vi "SCMP - Externally Triggered Image Acquisition - v5.vi"(0 "FPS":dbl=10.0 format="%.1g", 1 "LCVR Voltages":dbl[][](array[numeric]), 2 "Mod/Seq":bool, 5 "Cycles":i32=1 min=1 max=30 step=1, 7 "Save to FITS?":bool=TRUE, 9 "Headers In":T12[](array[typedef])=[{"Wavelength (nm)"=530.15, "Exposure (s)"=0.05, "Tuning Delay (ms)"=1000.0, "Beam Type (-1/1)"=1.0, "Tuning Voltages"=[1.111, 2.222, 3.333, 4.444], "Observer"="observer", "Light Shapping Diffuser"=enum."In Beam", "Comment"="", "Data Type"=9, "Mod Cycles"=0, "SCD Calibration Optics"=enum."1 - Polarizer @0, I+Q", "SCD Emission Line Filter"=enum."1-557.6nm", "Cookbook"="", "COMP-S Calibration Wheel"=enum."Dark", "COMP-S Andover Filter Wheel"=enum."530.3nm/HWB 0.34nm (Fe XIV)", "FOV Rotation (deg)"=66.0, "Objective Lens Position (mm)"=0.0, "Occulter size"=0.0, "Time End"=timestamp(3382374145.421875 s since 1904-01-01), "Acc Exposure (s)"=0.0, "Time Stamp Array"=[], "Camera Serial Number"=[], "Camera Temp"=[], "Camera PI (mm)"=[], "Time Start"=timestamp(3382374145.421875 s since 1904-01-01), "Peripherals"={"ILX controler"=FALSE, "Zone temperatures"=FALSE, "Andor"=FALSE, "Andor 2"=FALSE, "PI Stages"=FALSE, "AISAS mechanisms"=FALSE, "AISAS Mech.lvclass"=refnum, "Zone temp ref"=variant, "FWs"=FALSE}, "FITS paths"=[], "Cameras"=enum."Andor", "load preset cbk"=FALSE, "periodic check count"=0, "COMP-S Calibration Wheel 2"=enum."Dark", "Calib"=enum."Dark", "Abso Aperture"=40.0, "Nominal Aperture"=196.0}] {"Nominal Aperture" format="%.1f"; "Abso Aperture" format="%.1f"; "Camera PI (mm)" format="%_3g"; "Acc Exposure (s)" format="%^.3g"; "Occulter size" format="%.2f"; "Objective Lens Position (mm)" min=70.0 max=152.0 format="%.2f"; "FOV Rotation (deg)" format="%.1f"; "Data Type" items=["LIVE", "DARK", "FLAT", "CALI", "OBSE", "ABSO", "AURE", "TARG", "OBJE", "HOLE", "OREX", "THRO", "CHIP"]; "Exposure (s)" format="%^.3g"; "Wavelength (nm)" format="%_6g"}, 11 "error in":errorcluster, 12 "Andor Neo":T13[](array[typedef]) {"Exposure (s)" format="%^.3g"; "Time at Synch" format="%<%H:%M:%S>T"; "Interframe Time" format="%#_3g"; "Frame Readout Time" format="%_3g"; "Row Readout Time" format="%_3g"}) -> (3 "FITS Path Out":path, 6 "Image":u32[][](array[numeric]), 8 "Camera R Image":u32[][](graph), 10 "Headers Out":T2[](array[typedef]) {"Nominal Aperture" format="%.1f"; "Abso Aperture" format="%.1f"; "Camera PI (mm)" format="%_3g"; "Acc Exposure (s)" format="%^.3g"; "Occulter size" format="%.2f"; "Objective Lens Position (mm)" min=70.0 max=152.0 format="%.2f"; "FOV Rotation (deg)" format="%.1f"; "Exposure (s)" format="%^.3g"; "Wavelength (nm)" format="%_6g"}, 13 "FITS Path Out 2":path, 14 "Break":bool, 15 "error out":errorcluster)   [LabVIEW 2014]
doc: "The LL Sequence VI acquires a sequence of images and displays them in an array of image controls using the low-level acquisition VIs. A sequence is appropriate for applications that process multiple images. You can configure a sequence to acquire every frame or to skip a variable number of frames between each image.\n\nTop Level Code Overview\n1) Initialize Camera (Global Shutter, High Well, Low Noise, exposure time, etc.)\n2) Create a buffer set equal in size to the # of trigger pulses (e.g. 100) which is the same as the # of expected images \n3) Start the camera acquisition THEN start the DAQmx task (use merge error cluster to gurantee this)"
uses:
  Camera/Andor Neo Info.ctl
  Controls/run cbk timeout.ctl
  <vilib>/Waveform/WDTOps.llb/WDT Waveform Duration DBL.vi
  <vilib>/DAQmx/write.llb/DAQmx Write (Analog 1D Wfm NChan NSamp).vi
  <vilib>/DAQmx/create/channels.llb/DAQmx Create Channel (AO-Voltage-Basic).vi
  <vilib>/DAQmx/configure/timing.llb/DAQmx Timing (Use Waveform).vi
  Controls/Global demo.vi
  Controls/beaning.ctl
  Controls/SCD - Calibration Optics Filter Wheel.ctl
  AISAS/Controls/Diffuser.ctl
  Controls/SCD - FITS Cluster.ctl
  Controls/SCD - EDT - Emission Line Filter Wheel.ctl
  Controls/CoMP-S Controls/Polarization Optics Filter Wheel.ctl
  Controls/CoMP-S Controls/Emission Line Filter Wheel.ctl
  AISAS/Controls/focus.ctl
  AISAS/Mech/AISAS Mech.lvclass
  Controls/peripherals.ctl
  Controls/Cameras select.ctl
  Controls/FITS Data type.ctl
panel:
  out "Break 2":bool
  out "display refresh":bool
  out "seq cycles":i32=1
  out "error dequeue RAM":errorcluster
  out "mod cycles *4":i32=1
  out "error cam dequeue & queue RAM":errorcluster
  out "error dequeue 2":errorcluster
  in  "count 2":i32
  in  "Tab Control":T1(tab)
  out "Camera T Image":u32[][](graph)
  out "# elements in RAM queue":i32
  out "Image Acq (s)":dbl(slide)=4151.832132564842
  out "Image SSD Saving":i32(slide) scale=0.0..1.0
  in  "user break":bool
  out "Camera T Image wide":u32[][](graph)
  out "# images to acquire":i32
  out "Image Acq Started":bool
  out "PixelData [U16]":u16[](array[numeric])
  out "ByteData [U8]":u8[](array[numeric])
  in  "image pointers":u64[](array[numeric])
  in  "imageNo":i32
  in  "count":i32
  out "# wavelengths":i32=1
  out "Exposure Get (s)":dbl=0.09 format="%_3p"
  out "# elements in queue":i32
  out "Image Cam":u32[][](graph)
  out "# buffer":i32
  in  "image pointers 2":u64[](array[numeric])
  in  "imageNo 2":i32
  out "# elements in queue 2":i32
  out "# buffer 2":i32
  out "Image transfering":u32(slide) scale=0.0..40.0
  out "Acquisition Estimate (s)":dbl format="%0.2f"
  out "Image Acq":i32(slide) scale=0.0..40.0
  out "Image Acq 2":i32(slide) scale=0.0..40.0
  out "Image SSD Saving 2":i32(slide) scale=0.0..1.0
  out "Time Start":timestamp=timestamp(3382374145.421875 s since 1904-01-01) format="%<%H:%M:%S%3u\n%x>T"
  out "Time stamp arr":timestamp[](array[timestamp]) format="%<%H:%M:%S%3u>T"
  out "COMP Waveforms":waveform(dbl)[](graph)
  out "SCD Waveforms":waveform(dbl)[](graph)
  out "Time stamp arr 2":timestamp[](array[timestamp]) format="%<%H:%M:%S%3u>T"
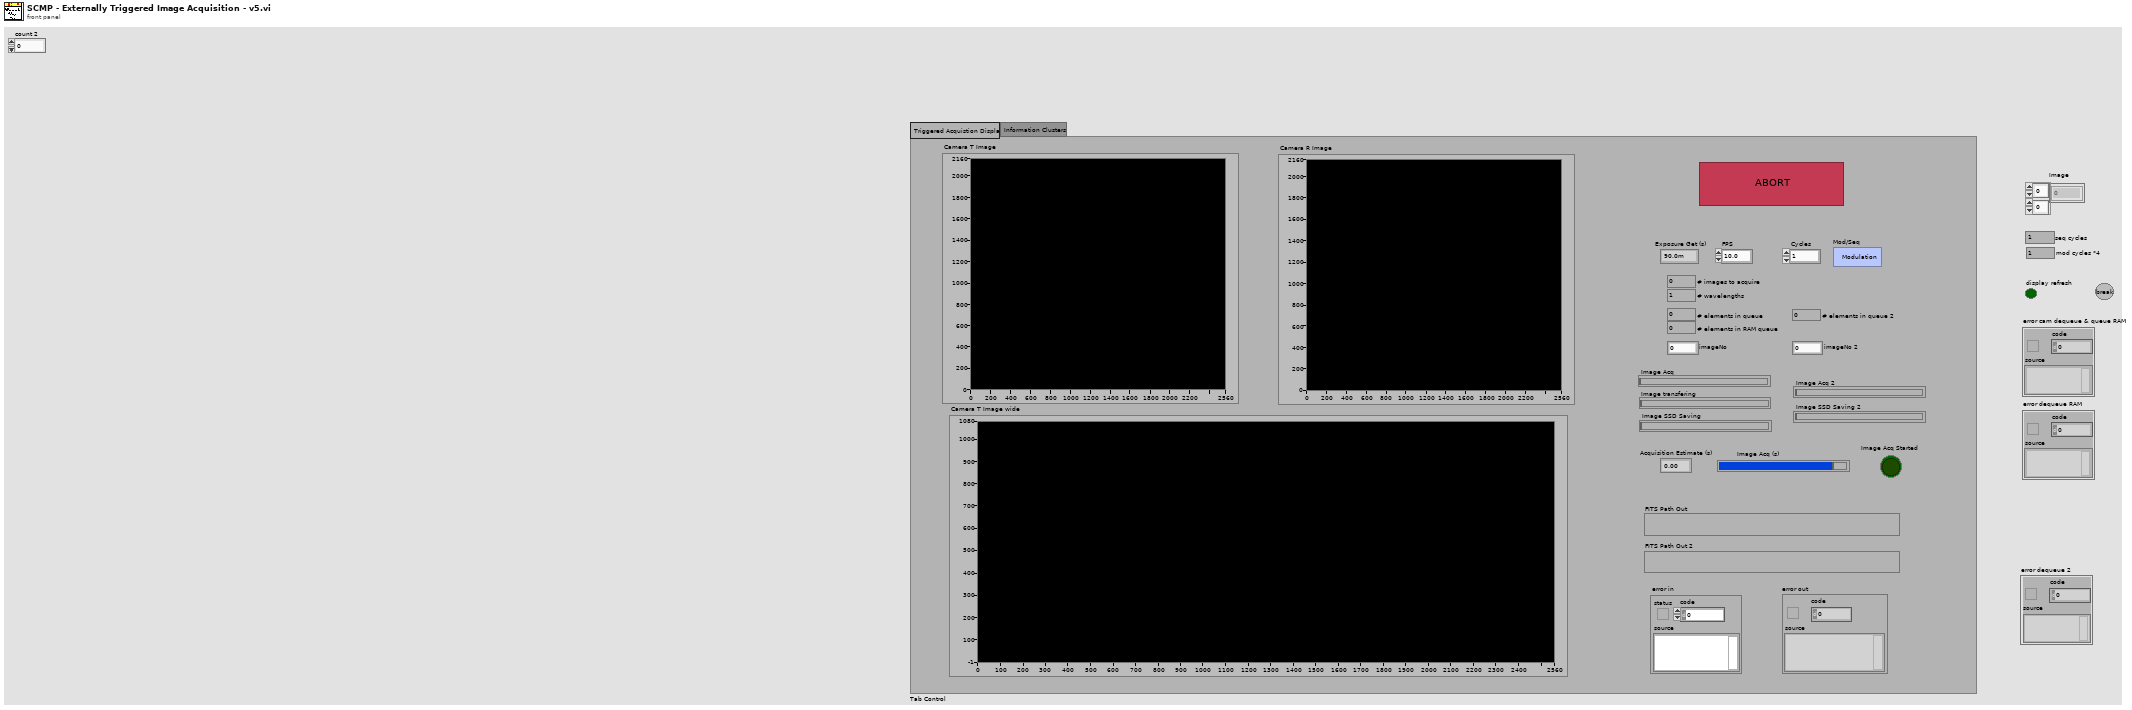
[diagram p1: front panel]
types:
  T1 = enum32{"Triggered Acquistion Display", "Information Clusters"}
  T2 = typedef "SCD - FITS Cluster.ctl" = cluster{"Wavelength (nm)":dbl, "Exposure (s)":dbl, "Tuning Delay (ms)":dbl, "Beam Type (-1/1)":dbl, "Tuning Voltages":dbl[], "Observer":string, "Light Shapping Diffuser":T3, "Comment":string, "Data Type":T4, "Mod Cycles":u16, "SCD Calibration Optics":T5, "SCD Emission Line Filter":T6, "Cookbook":string, "COMP-S Calibration Wheel":T7, "COMP-S Andover Filter Wheel":T8, "FOV Rotation (deg)":dbl, "Objective Lens Position (mm)":T9, "Occulter size":dbl, "Time End":timestamp, "Acc Exposure (s)":dbl, "Time Stamp Array":timestamp[], "Camera Serial Number":string[], "Camera Temp":dbl[], "Camera PI (mm)":dbl[], "Time Start":timestamp, "Peripherals":T10, "FITS paths":path[], "Cameras":T11, "load preset cbk":bool, "periodic check count":i32, "COMP-S Calibration Wheel 2":T7, "Calib":enum16{"Dark", "Flat"}, "Abso Aperture":dbl, "Nominal Aperture":dbl, "Pointer IP":string}
  T3 = typedef "Diffuser.ctl" = enum16{"Out of Beam", "In Beam"}
  T4 = typedef "FITS Data type.ctl" = enum16{"LIVE", "DARK", "FLAT", "CALI", "OBSE", "ABSO", "AURE", "TARG", "OBJE", "HOLE", "OREX", "THRO", "CHIP"}
  T5 = typedef "SCD - Calibration Optics Filter Wheel.ctl" = enum16{"1 - Polarizer @0, I+Q", "2 - Polarizer @90, I-Q", "3 - Polarizer @45, I+U", "4 - Polarizer @135, I-U", "5 - Polarizer @0, Retarder @45, I+V", "6 - Polarizer @0, Retarder @135, I-V", "7 - Dark", "8 - Clear", "9 - N/A"}
  T6 = typedef "SCD - EDT - Emission Line Filter Wheel.ctl" = enum16{"1-557.6nm", "2-587.6nm", "3-589.6nm", "4-630.2nm", "5-656.4nm", "6-849.8nm", "7-854.2nm", "8-866.2nm", "9-1083.0nm"}
  T7 = typedef "Polarization Optics Filter Wheel.ctl" = enum16{"Dark", "Clear", "Exchange Lens", "Polarizer @0, I+Q", "Polarizer @90, I-Q", "Polarizer @45, I+U", "Polarizer @135, I-U", "Polarizer @0, Retarder @45, I+V", "Polarizer @0, Retarder @135, I-V"}
  T8 = typedef "Emission Line Filter Wheel.ctl" = enum16{"530.3nm/HWB 0.34nm (Fe XIV)", "587.6nm/HBW 0.44nm (He I D3)", "637.5nm/HBW 0.53nm (Fe X)", "656.3nm/HBW 0.57nm (H-Alpha)", "789.2nm/HBW 0.85nm (Fe XI)", "854.2nm/HBW 1.01nm (Ca I)", "1074.7nm/HBW 2.34nm (Fe XIII)", "1079.8nm/HBW 1.64nm (Fe XIII)", "1083.0nm/HBW 1.66nm (He I)"}
  T9 = typedef "focus.ctl" = dbl
  T10 = typedef "peripherals.ctl" = cluster{"ILX controler":bool, "Zone temperatures":bool, "Andor":bool, "Andor 2":bool, "PI Stages":bool, "AISAS mechanisms":bool, "AISAS Mech.lvclass":refnum<class "AISAS Mech.lvclass">, "Zone temp ref":variant, "FWs":bool}
  T11 = typedef "Cameras select.ctl" = enum16{"Andor", "GDR"}
  T12 = typedef "SCD - FITS Cluster.ctl" = cluster{"Wavelength (nm)":dbl, "Exposure (s)":dbl, "Tuning Delay (ms)":dbl, "Beam Type (-1/1)":dbl, "Tuning Voltages":dbl[], "Observer":string, "Light Shapping Diffuser":T3, "Comment":string, "Data Type":u16, "Mod Cycles":u16, "SCD Calibration Optics":T5, "SCD Emission Line Filter":T6, "Cookbook":string, "COMP-S Calibration Wheel":T7, "COMP-S Andover Filter Wheel":T8, "FOV Rotation (deg)":dbl, "Objective Lens Position (mm)":T9, "Occulter size":dbl, "Time End":timestamp, "Acc Exposure (s)":dbl, "Time Stamp Array":timestamp[], "Camera Serial Number":string[], "Camera Temp":dbl[], "Camera PI (mm)":dbl[], "Time Start":timestamp, "Peripherals":T10, "FITS paths":path[], "Cameras":T11, "load preset cbk":bool, "periodic check count":i32, "COMP-S Calibration Wheel 2":T7, "Calib":enum16{"Dark", "Flat"}, "Abso Aperture":dbl, "Nominal Aperture":dbl}
  T13 = typedef "Andor Neo Info.ctl" = cluster{"Handle":i32, "Pixel Encoding":string, "AOI Width":i32, "AOI Height":i32, "AOI Stride":i32, "Row Readout Time":dbl, "Frame Readout Time":dbl, "Interframe Time":dbl, "Semaphore":T14, "SerialNumber":string, "Camera Model":string, "Controller ID":string, "Firmware Version":string, "Shutter":string, "BDiv":u8, "Time at Synch":timestamp, "Idx":i32, "PreAmp":string, "Binning":T15, "PixelReadoutRate":string, "Exposure (s)":dbl, "Image Bytes":i64, "Image Pixels":i64, "SpuriousNoiseFilter":bool, "Overlap":bool, "CycleMode":string}
  T14 = typedef "Semaphore RefNum" = refnum<k1>
  T15 = typedef "beaning.ctl" = enum16{"1x1", "2x2", "3x3", "4x4", "8x8"}
  T16 = enum8{"Enabled", "Disabled", "Disabled and Grayed Out"}
  T17 = typedef "run cbk timeout.ctl" = i32
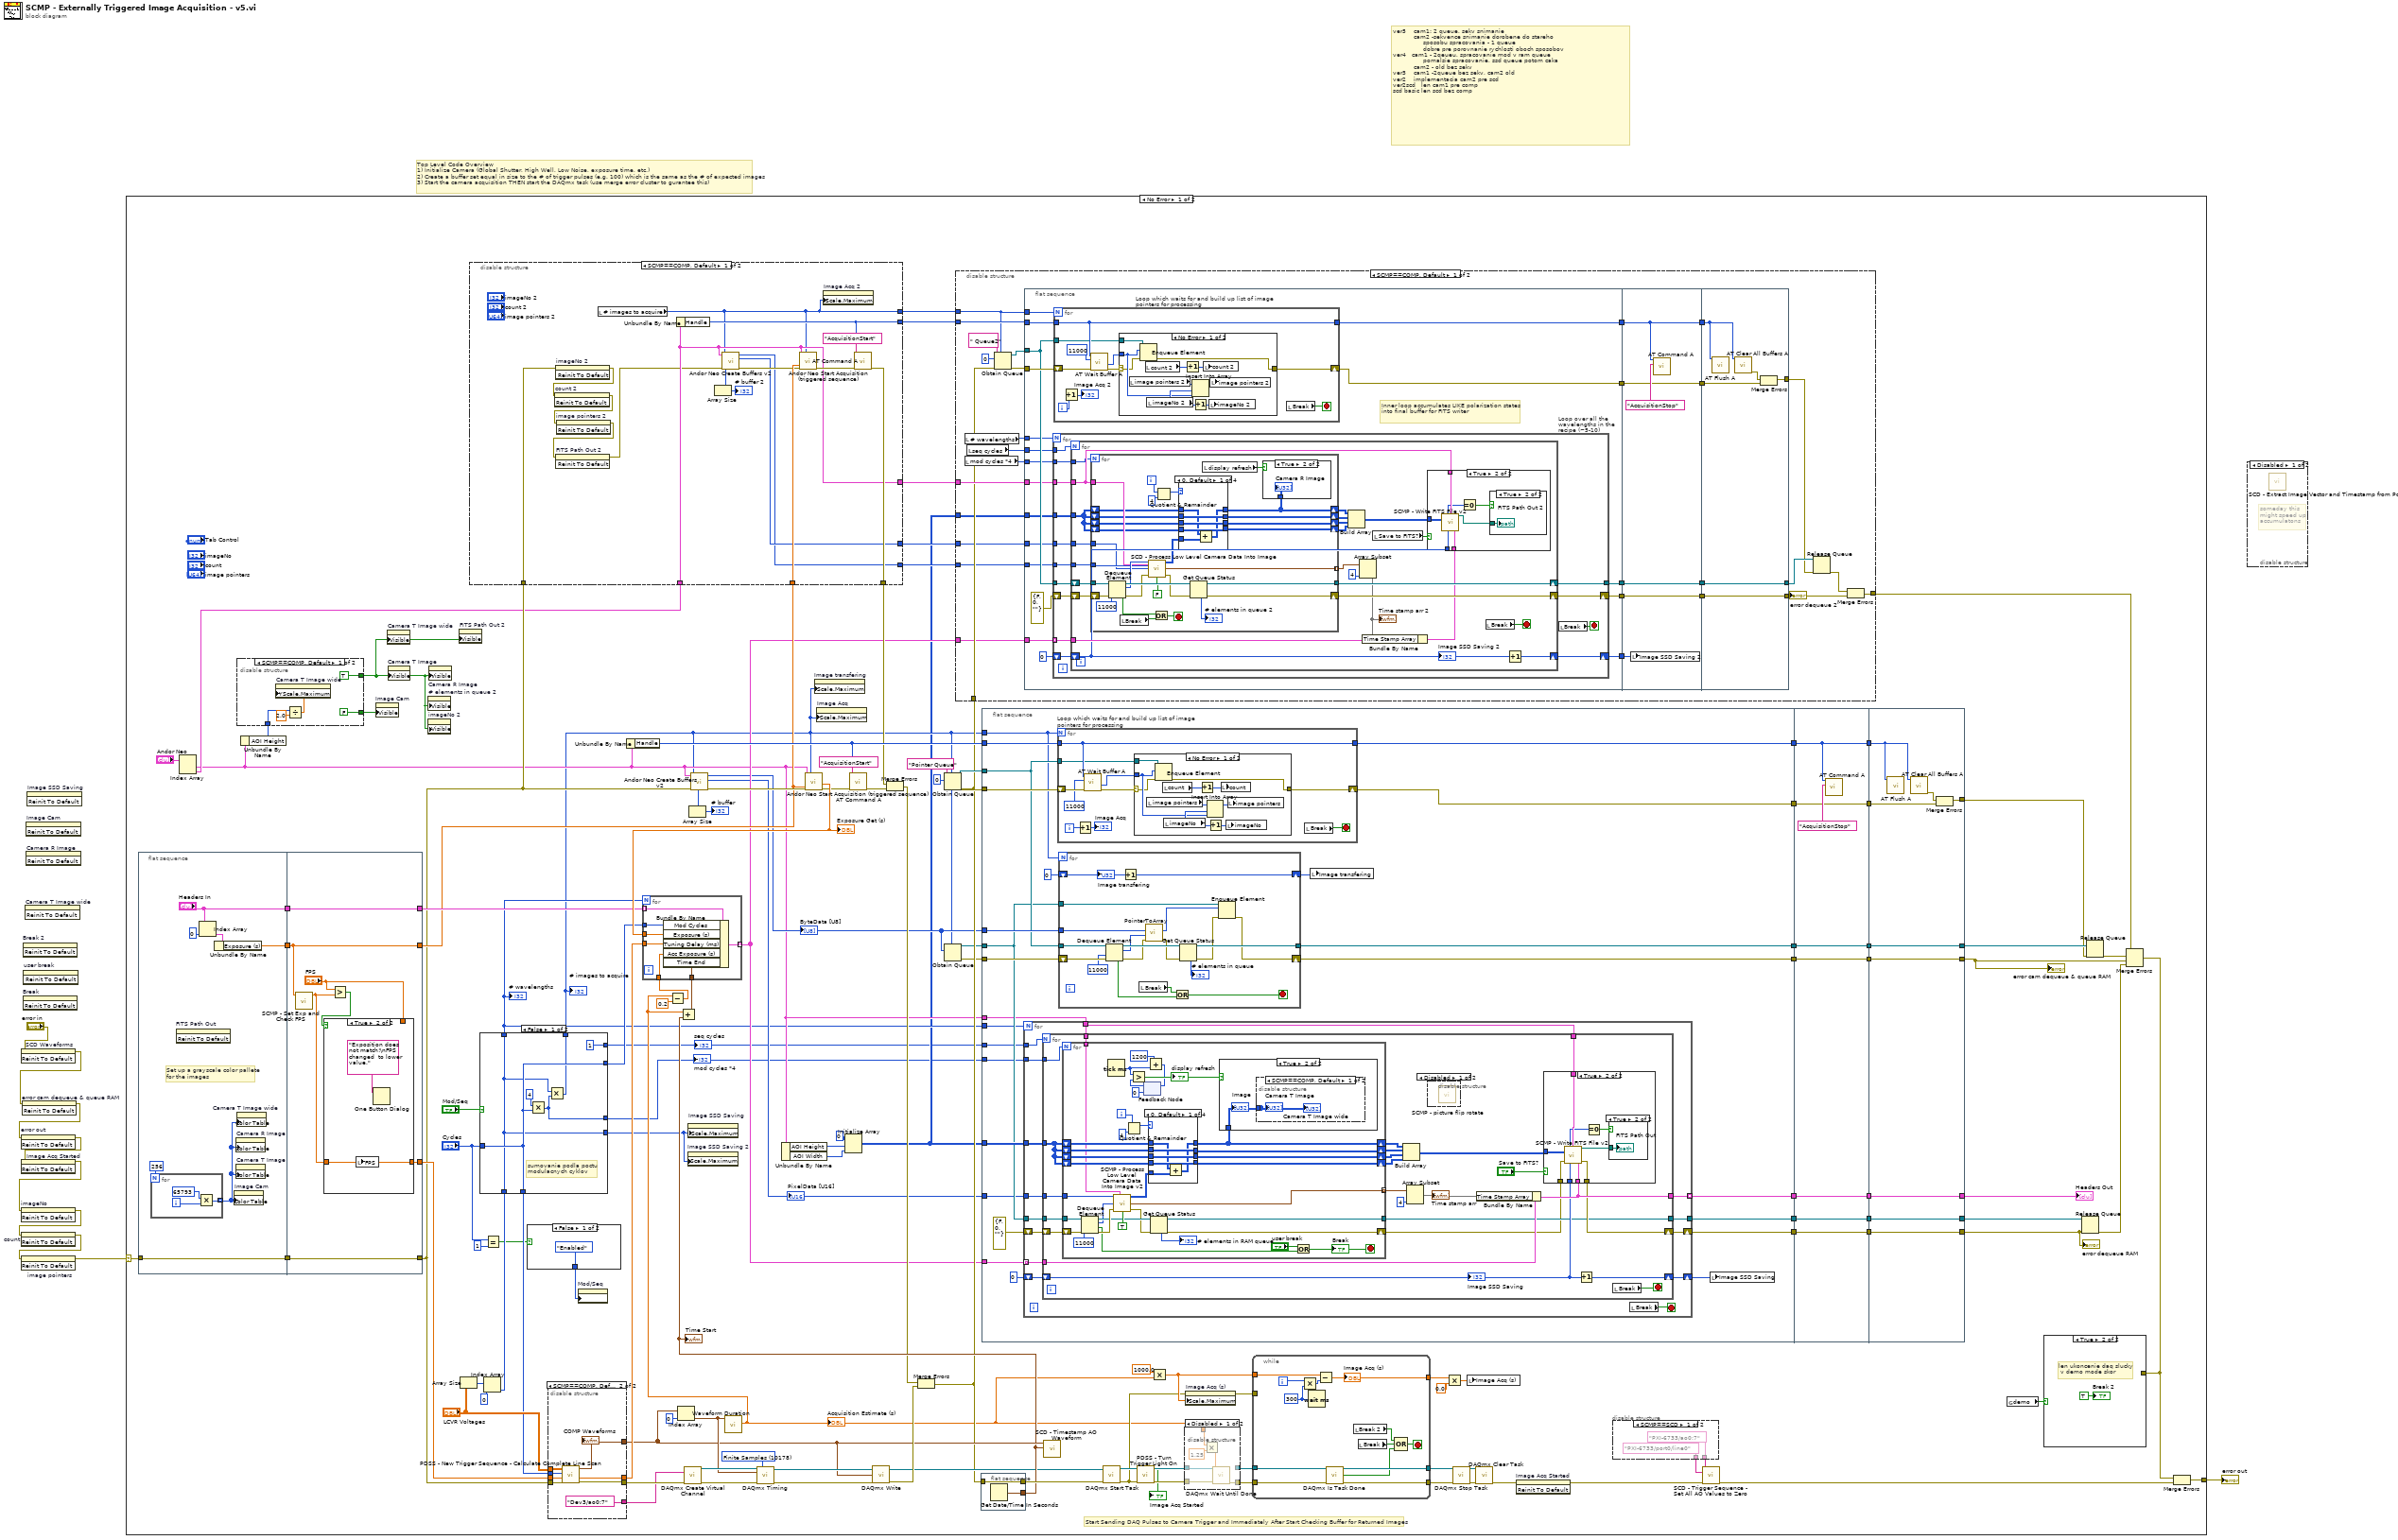
[diagram p0: block diagram]
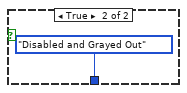
[diagram p3: hidden frame]
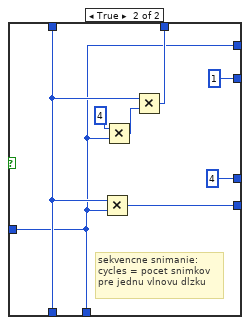
[diagram p6: hidden frame]
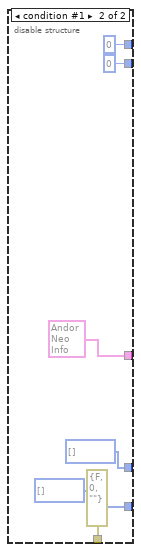
[diagram p7: hidden frame]
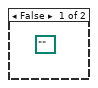
[diagram p8: hidden frame]
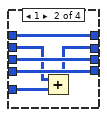
[diagram p11: hidden frame]
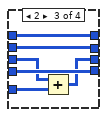
[diagram p12: hidden frame]
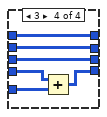
[diagram p13: hidden frame]
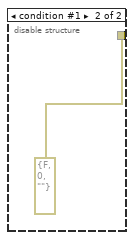
[diagram p15: hidden frame]
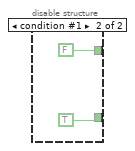
[diagram p17: hidden frame]
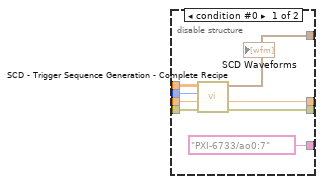
[diagram p18: hidden frame]
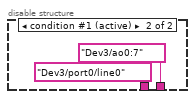
[diagram p19: hidden frame]
diagram:
  # "ver5    cam1: 2 queue, sekv snimanie\n           cam2 -sekvence snimanie dorobene do stareho \n                sposobu spracovania - 1 queue \n                dobre pre porovnanie rychlosti oboch sposobov\nver4   cam1 - 2qeueu, spracovanie mod v ram queue\n                pomalsie spracovanie, ssd queue potom caka\n           cam2 - old bez sekv\nver3    cam1 -2queue bez sekv, cam2 old\nver2    implementacia cam2 pre scd\nver2scd   len cam1 pre comp\nscd basic len scd bez comp"
  # "Top Level Code Overview\n1) Initialize Camera (Global Shutter, High Well, Low Noise, exposure time, etc.)\n2) Create a buffer set equal in size to the # of trigger pulses (e.g. 100) which is the same as the # of expected images \n3) Start the camera acquisition THEN start the DAQmx task (use merge error cluster to gurantee this)"
  n1 = invoke on="SCD Waveforms" class="WFGraph (strict)" method="Reinit To Default"(error in="error in") -> (error out=w3:errorcluster)  [unwired: 2 in, 2 out]
  n2 = invoke on="error cam dequeue & queue RAM" class="Clust (strict)" method="Reinit To Default"(error in=w3) -> (error out=w2:errorcluster)  [unwired: 2 in, 2 out]
  n3 = invoke on="error out" class="Clust (strict)" method="Reinit To Default"(error in=w2) -> (error out=w8:errorcluster)  [unwired: 2 in, 2 out]
  n4 = invoke on="Image Acq Started" class="Bool (strict)" method="Reinit To Default"(error in=w8) -> (error out=w4:errorcluster)  [unwired: 2 in, 2 out]
  n5 = invoke on="imageNo" class="DigNum (strict)" method="Reinit To Default"(error in=w4) -> (error out=w7:errorcluster)  [unwired: 2 in, 2 out]
  n6 = invoke on="count" class="DigNum (strict)" method="Reinit To Default"(error in=w7) -> (error out=w6:errorcluster)  [unwired: 2 in, 2 out]
  n7 = invoke on="image pointers" class="Arr (strict)" method="Reinit To Default"(error in=w6) -> (error out=w5:errorcluster)  [unwired: 2 in, 2 out]
  n8 = invoke on="Break 2" class="Bool (strict)" method="Reinit To Default"() -> ()  [unwired: 3 in, 3 out]
  n9 = invoke on="Break" class="Bool (strict)" method="Reinit To Default"() -> ()  [unwired: 3 in, 3 out]
  n10 = invoke on="user break" class="Bool (strict)" method="Reinit To Default"() -> ()  [unwired: 3 in, 3 out]
  n11 = invoke on="Camera T Image wide" class="IntGraph (strict)" method="Reinit To Default"() -> ()  [unwired: 3 in, 3 out]
  n12 = invoke on="Image Cam" class="IntGraph (strict)" method="Reinit To Default"() -> ()  [unwired: 3 in, 3 out]
  n13 = invoke on="Camera R Image" class="IntGraph (strict)" method="Reinit To Default"() -> ()  [unwired: 3 in, 3 out]
  n14 = invoke on="Image SSD Saving" class="Slide (strict)" method="Reinit To Default"() -> ()  [unwired: 3 in, 3 out]
  n15 = case shown="No Error" w5 {
    selector: w5 -> [w85 w627]
    tunnel: [w111 w627] -> w9
    frame No Error {
      w134 = 10178 items=["Finite Samples"=10178, "Continuous Samples"=10123] ("sample mode")
      # "Start Sending DAQ Pulses to Camera Trigger and Immediately After Start Checking Buffer for Returned Images"
      n16 = flat-sequence {
        tunnel: w85 -> [w383]
        tunnel: [w383] -> w77
        tunnel: ["Headers In"] -> w75
        tunnel: [w379] -> w74
        tunnel: [w394] -> w56
        tunnel: w77 -> [w394]
        tunnel: [w393] -> w76
        tunnel: w75 -> [w393]
        tunnel: [w388] -> w66
        tunnel: w74 -> [w388]
        tunnel: [w391] -> w73
        frame #0 {
          # "Set up a grayscale color pallete for the images"
          n17 = for {
            N: 256 -> [_]
            tunnel: [w386] -> w378 mode=indexing
            i -> [w387]
            n18 = Multiply(x=65793, y=w387) -> (x*y=w386:i32)
          }
          n19 = invoke on="FITS Path Out" class="Path" method="Reinit To Default"() -> ()  [unwired: 3 in, 3 out]
          n20 = Index Array(array="Headers In", index=0) -> (element=w381:T12)
          n21 = Unbundle By Name(w381) -> ("Exposure (s)"=w379:dbl)
          n22 = property on="Image Cam" class="IntGraph (strict)"("Color Table"=w378) -> ()  [unwired: 2 in, 2 out]
          n23 = property on="Camera R Image" class="IntGraph (strict)"("Color Table"=w378) -> ()  [unwired: 2 in, 2 out]
          n24 = property on="Camera T Image" class="IntGraph (strict)"("Color Table"=w378) -> ()  [unwired: 2 in, 2 out]
          n25 = property on="Camera T Image wide" class="IntGraph (strict)"("Color Table"=w378) -> ()  [unwired: 2 in, 2 out]
        }
        frame #1 {
          n26 = call "SCMP - Set Exp and Check FPS.vi"("Exposure [s]"=w388) -> ("FPS"=w389:dbl)  [unwired: 9 in, 1 out]
          n27 = Greater?(x="FPS", y=w389) -> (0:w392:bool)
          n28 = case shown="True" w392 {
            tunnel: [w395 w396] -> w391
            tunnel: "FPS" -> [w395 _]
            tunnel: w389 -> [_ w396]
            frame False {
            }
            frame True {
              n29 = local write "FPS"(w396) -> ()
              n30 = One Button Dialog(message="Exposition does not match!\nFPS changed  to lower value.") -> ()  [unwired: 1 in, 1 out]
            }
          }
        }
      }
      n31 = Index Array(array="Andor Neo") -> (element #1=w19:T13, element #2=w54:T13)  [unwired: 2 in]
      n32 = Unbundle By Name(w19) -> ("AOI Height"=w92:i32)
      n33 = disable-structure shown="SCMP==COMP, Default" {
        disable-tunnel: w92 -> [w401 _]
        disable-tunnel: [TRUE ("Visible") FALSE ("Visible")] -> w22
        disable-tunnel: [FALSE ("Visible") TRUE ("Visible")] -> w91
        frame condition #0 (active) {
          n34 = Divide(x=w401, y=2.0) -> (x/y=w402:dbl)
          n35 = property on="Camera T Image wide" class="IntGraph (strict)"("YScale.Maximum"=w402) -> ()  [unwired: 2 in, 2 out]
        }
        frame condition #1 {
        }
      }
      n36 = property on="Image Cam" class="IntGraph (strict)"("Visible"=w91) -> ()  [unwired: 2 in, 2 out]
      n37 = property on="Camera T Image wide" class="IntGraph (strict)"("Visible"=w22) -> ()  [unwired: 2 in, 2 out]
      n38 = property on="Camera T Image" class="IntGraph (strict)"("Visible"=w22) -> ()  [unwired: 2 in, 2 out]
      n39 = property on="# elements in queue 2" class="DigNum (strict)"("Visible"=w22) -> ()  [unwired: 2 in, 2 out]
      n40 = property on="imageNo 2" class="DigNum (strict)"("Visible"=w22) -> ()  [unwired: 2 in, 2 out]
      n41 = property on="Camera R Image" class="IntGraph (strict)"("Visible"=w22) -> ()  [unwired: 2 in, 2 out]
      n42 = property on="FITS Path Out 2" class="Path"("Visible"=w22) -> ()  [unwired: 2 in, 2 out]
      n43 = Array Size(array="LCVR Voltages") -> (size(s)=w120:i32[])
      n44 = disable-structure shown="SCMP==COMP, Default" {
        disable-tunnel: w66 -> [w189 _]
        disable-tunnel: [w188 errorcluster {"status"=FALSE, "code"=0, "source"=""} ("error out")] -> w63
        disable-tunnel: [w182 0 ("Handle")] -> w60
        disable-tunnel: [w181 i64[] [] ("PixelData")] -> w59
        disable-tunnel: [w180 u8[] [] ("ByteData")] -> w58
        disable-tunnel: [w173 0 ("# images to acquire")] -> w57
        disable-tunnel: w56 -> [w176 _]
        disable-tunnel: [w179 T13 {"Handle"=0, "Pixel Encoding"="", "AOI Width"=0, "AOI Height"=0, "AOI Stride"=0, "Row Readout Time"=0.0, "Frame Readout Time"=0.0, "Interframe Time"=0.0, "Semaphore"=refnum, "SerialNumber"="", "Camera Model"="", "Controller ID"="", "Firmware Version"="", "Shutter"="Global", "BDiv"=1, "Time at Synch"=timestamp(3029526000.379448 s since 1904-01-01), "Idx"=0, "PreAmp"="", "Binning"=enum."1x1", "PixelReadoutRate"="", "Exposure (s)"=0.05, "Image Bytes"=0, "Image Pixels"=0, "SpuriousNoiseFilter"=FALSE, "Overlap"=FALSE, "CycleMode"=""} ("Neo Info")] -> w55
        disable-tunnel: w54 -> [w179 _]
        frame condition #0 (active) {
          n45 = invoke on="imageNo 2" class="DigNum (strict)" method="Reinit To Default"(error in=w176) -> (error out=w178:errorcluster)  [unwired: 2 in, 2 out]
          n46 = invoke on="count 2" class="DigNum (strict)" method="Reinit To Default"(error in=w178) -> (error out=w177:errorcluster)  [unwired: 2 in, 2 out]
          n47 = invoke on="image pointers 2" class="Arr (strict)" method="Reinit To Default"(error in=w177) -> (error out=w175:errorcluster)  [unwired: 2 in, 2 out]
          n48 = invoke on="FITS Path Out 2" class="Path" method="Reinit To Default"(error in=w175) -> (error out=w174:errorcluster)  [unwired: 2 in, 2 out]
          n49 = local read "# images to acquire"() -> (w173:i32)
          n50 = Unbundle By Name(w179) -> ("Handle"=w182:i32)
          n51 = call "Andor Neo Create Buffers v2.vi"("error in"=w174, "Number of Images"=w173, "Camera Info"=w179) -> ("error out"=w186:errorcluster, "PixelData"=w181:i64[], "ByteData"=w180:u8[], "# of Andor buffers"=w184:i32)  [unwired: 4 in, 1 out]
          n52 = Array Size(array=w184) -> (size(s)=→"# buffer 2":i32)
          n53 = call "Andor Neo Start Acquisition (triggered sequence).vi"("Exposure Set (s)"=w189, "error in"=w186, "Frames"=w173, "Camera Info"=w179) -> ("error out"=w185:errorcluster)  [unwired: 6 in, 1 out]
          n54 = property on="Image Acq 2" class="Slide (strict)"("Scale.Maximum"=w173) -> ()  [unwired: 2 in, 2 out]
          n55 = call <userlib>:"AT Command A.vi"("error in (no error)"=w185, "Feature"="AcquisitionStart" ("Command"), "Handle"=w182) -> ("error out"=w188:errorcluster)  [unwired: 7 in, 1 out]
        }
        frame condition #1 {
        }
      }
      n56 = Index Array(array=w120, index=0) -> (element=w37:i32)
      n57 = case shown="False" "Mod/Seq" {
        tunnel: [w150 4] -> w12
        tunnel: [w148 w157] -> w14
        tunnel: [w146 w154] -> w15
        tunnel: w37 -> [w146 w154]
        tunnel: [w149 1 ("Cycles")] -> w39
        tunnel: [w149 w152] -> w38
        tunnel: "Cycles" -> [w149 w152]
        tunnel: [w146 w153] -> w10
        tunnel: [1 ("value") w152] -> w11
        frame False {
          # "sumovanie podla poctu\nmodulacnych cyklov"
          n58 = Multiply(x=4 ("value"), y=w149) -> (x*y=w150:i32)
          n59 = Multiply(x=w146, y=w150) -> (x*y=w148:i32)
        }
        frame True {
          # "sekvencne snimanie:\ncycles = pocet snimkov\npre jednu vlnovu dlzku"
          n60 = Multiply(x=w154, y=w152) -> (x*y=w153:i32)
          n61 = Multiply(x=4 ("value"), y=w152) -> (x*y=w158:i32)
          n62 = Multiply(x=w154, y=w158) -> (x*y=w157:i32)
        }
      }
      "# wavelengths" <- w15
      "# images to acquire" <- w14
      "mod cycles *4" <- w12
      "seq cycles" <- w11
      n63 = Equal?(x="Cycles", y=1) -> (x = y?=w24:bool)
      n64 = case shown="False" w24 {
        tunnel: [T16."Enabled" ("Disabled") T16."Disabled and Grayed Out" ("Disabled")] -> w23
        frame False {
        }
        frame True {
        }
      }
      n65 = disable-structure shown="SCMP==COMP, Default" {
        disable-tunnel: [w412 w416] -> w127
        disable-tunnel: "LCVR Voltages" -> [w411 w420]
        disable-tunnel: [w406 w414] -> w97
        disable-tunnel: w73 -> [w410 w418]
        disable-tunnel: w56 -> [w409 w417]
        disable-tunnel: [w408 w415] -> w98
        disable-tunnel: w38 -> [w407 w419]
        disable-tunnel: [tag "PXI-6733/ao0:7" ("physical channels") tag "Dev3/ao0:7" ("physical channels")] -> w71
        frame condition #0 {
          n66 = call "SCD - Trigger Sequence Generation - Complete Recipe.vi"("error in"=w409, "FPS"=w410, "Modulation Cycles\nAt Each Wavelength"=w407, "LCVR Voltages"=w411) -> ("error out"=w412:errorcluster, "LCVR Relaxtion Time"=w408:dbl, "SCD Waveforms (Graph)"=w406:waveform(dbl)[])  [unwired: 5 in]
          "SCD Waveforms" <- w406
        }
        frame condition #1 (active) {
          n67 = call "PDSS - New Trigger Sequence - Calculate Complete Line Scan.vi"("error in"=w417, "FPS"=w418, "Modulation Cycles\nAt Each Wavelength"=w419, "LCVR Voltages"=w420) -> ("error out"=w416:errorcluster, "LCVR Relaxtion Time"=w415:dbl, "AO Graph"=w414:waveform(dbl)[])  [unwired: 5 in]
          "COMP Waveforms" <- w414
        }
      }
      n68 = property on="Mod/Seq" class="Bool (strict)"("DisabledEnum"=w23) -> ()  [unwired: 2 in, 2 out]
      n69 = Unbundle By Name(w19) -> ("Handle"=w68:i32)
      n70 = Index Array(array=w97, index=0) -> (element=w124:waveform(dbl))
      n71 = call-poly <vilib>:"DAQmx Create Virtual Channel.vi"("physical channels"=w71, "error in"=w127) -> ("task out"=w132:refnum<k21>, "error out"=w133:errorcluster)  [unwired: 12 in]
      n72 = property on="Image SSD Saving 2" class="Slide (strict)"("Scale.Maximum"=w10) -> ()  [unwired: 2 in, 2 out]
      n73 = property on="Image SSD Saving" class="Slide (strict)"("Scale.Maximum"=w10) -> ()  [unwired: 2 in, 2 out]
      n74 = call "Andor Neo Create Buffers v2.vi"("error in"=w56, "Number of Images"=w14, "Camera Info"=w19) -> ("error out"=w110:errorcluster, "PixelData"=w16:i64[], "ByteData"=w21:u8[], "# of Andor buffers"=w84:i32)  [unwired: 4 in, 1 out]
      "ByteData [U8]" <- w21
      "PixelData [U16]" <- w16
      n75 = Array Size(array=w84) -> (size(s)=→"# buffer":i32)
      n76 = call-poly <vilib>:"Waveform Duration.vi"("waveform in"=w124) -> ("duration"=w34:dbl)  [unwired: 8 in, 2 out]
      "Acquisition Estimate (s)" <- w34
      n77 = Subtract(x=w34, y=0.2) -> (x-y=w86:dbl)
      n78 = Add(x=w34, y=w72) -> (x+y=w90:timestamp)
      n79 = call-poly <vilib>:"DAQmx Timing.vi"("task/channels in"=w132, "sample mode"=w134, "waveform"=w124, "error in"=w133) -> ("task out"=w125:refnum<k21>, "error out"=w126:errorcluster)  [unwired: 10 in]
      n80 = Unbundle By Name(w19) -> ("AOI Height"=w18:i32, "AOI Width"=w17:i32)
      n81 = call "Andor Neo Start Acquisition (triggered sequence).vi"("Exposure Set (s)"=w66, "error in"=w110, "Frames"=w14, "Camera Info"=w19) -> ("error out"=w88:errorcluster, "Exposure Get (s)"=w89:dbl)  [unwired: 6 in]
      "Exposure Get (s)" <- w89
      n82 = for {
        N: w15 -> [_]
        tunnel: [w431] -> w62 mode=indexing
        tunnel: w89 -> [w430]
        tunnel: w76 -> [w429] mode=indexing
        tunnel: w98 -> [w428]
        tunnel: w39 -> [w427]
        tunnel: w86 -> [w426]
        tunnel: w90 -> [w425]
        n83 = Bundle By Name(cluster=w429, "Mod Cycles"=w427, "Exposure (s)"=w430, "Tuning Delay (ms)"=w428, "Acc Exposure (s)"=w426, "Time End"=w425) -> (w431:T12)
      }
      n84 = property on="Image transfering" class="Slide (strict)"("Scale.Maximum"=w14) -> ()  [unwired: 2 in, 2 out]
      n85 = property on="Image Acq" class="Slide (strict)"("Scale.Maximum"=w14) -> ()  [unwired: 2 in, 2 out]
      n86 = Initialize Array(u32 0, w18, w17) -> (w13:u32[][])
      n87 = call <userlib>:"AT Command A.vi"("error in (no error)"=w88, "Feature"="AcquisitionStart" ("Command"), "Handle"=w68) -> ("error out"=w109:errorcluster)  [unwired: 7 in, 1 out]
      n88 = call-poly <vilib>:"DAQmx Write.vi"("task/channels in"=w125, "data"=w97, "error in"=w126) -> ("task out"=w67:refnum<k21>, "error out"=w113:errorcluster)  [unwired: 10 in, 1 out]
      n89 = Merge Errors(w63, w109) -> (w64:errorcluster)
      n90 = Merge Errors(w64, w113) -> (w65:errorcluster)
      n91 = Obtain Queue(max queue size (-1, unlimited)=w14, name (unnamed)="Pointer Queue", element data type=u64 0 ("Output buffer"), error in (no error)=w65) -> (queue out=w104:refnum<queue>, error out=w105:errorcluster)  [unwired: 1 in, 1 out]
      n92 = Obtain Queue(max queue size (-1, unlimited)=w14, element data type=w21) -> (queue out=w20:refnum<queue>, error out=w48:errorcluster)  [unwired: 3 in, 1 out]
      n93 = disable-structure shown="SCMP==COMP, Default" {
        disable-tunnel: w55 -> [w216 _]
        disable-tunnel: w65 -> [w215 _]
        disable-tunnel: w62 -> [w214 _]
        disable-tunnel: [w213 errorcluster {"status"=FALSE, "code"=0, "source"=""} ("error IO")] -> w61
        disable-tunnel: w60 -> [w210 _]
        disable-tunnel: w59 -> [w209 _]
        disable-tunnel: w58 -> [w208 _]
        disable-tunnel: w57 -> [w205 _]
        disable-tunnel: w13 -> [w197 _]
        frame condition #0 (active) {
          n94 = local read "# wavelengths"() -> (w204:i32)
          n95 = local read "mod cycles *4"() -> (w201:i32)
          n96 = local read "seq cycles"() -> (w196:i32)
          n97 = Obtain Queue(max queue size (-1, unlimited)=w205, name (unnamed)=" Queue2", element data type=u64 0 ("Output buffer"), error in (no error)=w215) -> (queue out=w207:refnum<queue>, error out=w206:errorcluster)  [unwired: 1 in, 1 out]
          n98 = flat-sequence {
            tunnel: w206 -> [w243]
            tunnel: w210 -> [w242]
            tunnel: [w241] -> w224
            tunnel: [w232] -> w223
            tunnel: w216 -> [w236]
            tunnel: w209 -> [w237]
            tunnel: w208 -> [w239]
            tunnel: w207 -> [w240]
            tunnel: [w238] -> w222
            tunnel: w201 -> [w234]
            tunnel: [w235] -> w221
            tunnel: w205 -> [w231]
            tunnel: w214 -> [w230]
            tunnel: w204 -> [w229]
            tunnel: [w227] -> w200
            tunnel: w197 -> [w226]
            tunnel: w196 -> [w225]
            tunnel: w224 -> [w367]
            tunnel: w223 -> [w366]
            tunnel: w222 -> [w369]
            tunnel: w221 -> [w368]
            tunnel: [w367] -> w220
            tunnel: [w369] -> w219
            tunnel: [w368] -> w218
            tunnel: [w366] -> w217
            tunnel: w200 -> [w365]
            tunnel: [w376] -> w198
            tunnel: [w375] -> w199
            tunnel: w220 -> [w373]
            tunnel: w219 -> [w371]
            tunnel: w218 -> [w376]
            tunnel: w217 -> [w374]
            tunnel: [w371] -> w202
            frame #0 {
              # "Inner loop accumulates LIKE polarization states into final buffer for FITS writer"
              n99 = for "Loop over all the wavelengths in the recipe (~5-10)" {
                N: w229 -> [_]
                tunnel: w240 -> [w257]
                tunnel: w239 -> [w256]
                tunnel: [w255] -> w238
                tunnel: w237 -> [w254]
                tunnel: w236 -> [w253]
                tunnel: w234 -> [w252]
                shift-right: [w251] -> w235
                shift-left: errorcluster {"status"=FALSE, "code"=0, "source"=""} ("error out") -> [w250]
                tunnel: w230 -> [w249] mode=indexing
                shift-right: [w247] -> w227
                shift-left: 0 ("Image SSD Saving 2") -> [w248]
                tunnel: w226 -> [w246]
                tunnel: w225 -> [w245]
                stop <- w244 stop-if-true
                n100 = for {
                  N: w245 -> [_]
                  tunnel: w256 -> [w279]
                  tunnel: w254 -> [w277]
                  tunnel: w253 -> [w276]
                  tunnel: w252 -> [w275]
                  tunnel: w249 -> [w271]
                  tunnel: w246 -> [w267]
                  shift-right: [w278] -> w255
                  shift-left: w257 -> [w280]
                  shift-right: [w274] -> w251
                  shift-left: w250 -> [w273]
                  shift-right: [w268] -> w247
                  shift-left: w248 -> [w269]
                  stop <- w266 stop-if-true
                  n101 = for {
                    N: w275 -> [_]
                    tunnel: w280 -> [w318]
                    tunnel: w279 -> [w315]
                    tunnel: [w302] -> w278
                    tunnel: w277 -> [w314]
                    tunnel: w276 -> [w313]
                    shift-right: [w288] -> w265
                    shift-left: w267 -> [w307]
                    shift-right: [w306] -> w264
                    shift-left: w267 -> [w308]
                    shift-right: [w305] -> w263
                    shift-left: w267 -> [w309]
                    shift-right: [w304] -> w262
                    shift-left: w267 -> [w310]
                    shift-right: [w297] -> w274
                    shift-left: w273 -> [w295]
                    tunnel: [w294] -> w259 mode=indexing
                    i -> [w296]
                    stop <- w290 stop-if-true
                    n102 = Dequeue Element(queue=w318, timeout in ms (-1)=11000, error in (no error)=w295) -> (queue out=w317:refnum<queue>, element=w316:u64, timed out?=w292:bool, error out=w299:errorcluster)
                    n103 = local read "Break"() -> (w291:bool)
                    n104 = call "SCD - Process Low Level Camera Data Into Image.vi"("Pointer In"=w316, "Neo Info"=w313, "ByteData (U8)"=w315, "PixelData (U16)"=w314, "error in (no error)"=w299, "scmp demo pic"=FALSE) -> ("Image (I32)"=w303:u32[][], "Timestamp"=w294:timestamp, "error out"=w298:errorcluster)  [unwired: 7 in]
                    n105 = Or(x=w292, y=w291) -> (x .or. y?=w290:bool)
                    n106 = Quotient & Remainder(x=w296, y=4) -> (x-y*floor(x/y)=w311:i32)  [unwired: 1 out]
                    n107 = case shown="0, Default" w311 {
                      tunnel: w310 -> [w323 w330 w336 w339]
                      tunnel: w309 -> [w324 w331 w333 w342]
                      tunnel: w308 -> [w325 w327 w337 w343]
                      tunnel: w307 -> [w321 w328 w334 w340]
                      tunnel: [w320 w328 w334 w340] -> w288
                      tunnel: [w325 w326 w337 w343] -> w306
                      tunnel: [w324 w331 w332 w342] -> w305
                      tunnel: [w323 w330 w336 w338] -> w304
                      tunnel: w303 -> [w322 w329 w335 w341]
                      frame 0, Default {
                        n108 = Add(x=w321, y=w322) -> (x+y=w320:u32[][])
                      }
                      frame 1 {
                        n109 = Add(x=w327, y=w329) -> (x+y=w326:u32[][])
                      }
                      frame 2 {
                        n110 = Add(x=w333, y=w335) -> (x+y=w332:u32[][])
                      }
                      frame 3 {
                        n111 = Add(x=w339, y=w341) -> (x+y=w338:u32[][])
                      }
                    }
                    n112 = Get Queue Status(queue=w317, error in (no error)=w298) -> (queue out=w302:refnum<queue>, error out=w297:errorcluster, # elements in queue=→"# elements in queue 2":i32)  [unwired: 1 in, 5 out]
                    n113 = local read "display refresh"() -> (w289:bool)
                    n114 = case shown="True" w289 {
                      tunnel: w288 -> [_ w319]
                      frame False {
                      }
                      frame True {
                        "Camera R Image" <- w319
                      }
                    }
                  }
                  n115 = Build Array(w265, w264, w263, w262) -> (w261:u32[][][])
                  n116 = Array Subset(array=w259, length=4) -> (w258:timestamp[])  [unwired: 1 in]
                  "Time stamp arr 2" <- w258
                  n117 = Bundle By Name(cluster=w271, "Time Stamp Array"=w258) -> (w272:T12)
                  n118 = local read "Save to FITS?"() -> (w270:bool)
                  n119 = case shown="True" w270 {
                    tunnel: w272 -> [_ w286]
                    tunnel: w276 -> [_ w285]
                    tunnel: w269 -> [_ w284]
                    tunnel: w261 -> [_ w281]
                    frame False {
                      (unwired) path "" ("FITS Path Out")
                    }
                    frame True {
                      n120 = call "SCMP - Write FITS File v2.vi"("FITS Header"=w286, "Andor"=w285, "Data"=w281, "Image #"=w284) -> ("FITS Path Out"=w283:path)  [unwired: 9 in, 2 out]
                      n121 = Equal To 0?(x=w284) -> (x = 0?=w282:bool)
                      n122 = case shown="True" w282 {
                        tunnel: w283 -> [_ w287]
                        frame False {
                        }
                        frame True {
                          "FITS Path Out 2" <- w287
                        }
                      }
                    }
                  }
                  n123 = local read "Break"() -> (w266:bool)
                  n124 = Increment(x=w269) -> (x+1=w268:i32)
                  "Image SSD Saving 2" <- w269
                }
                n125 = local read "Break"() -> (w244:bool)
              }
              n126 = for "Loop which waits for and build up list of image pointers for processing" {
                N: w231 -> [_]
                tunnel: w242 -> [w350]
                tunnel: [w350] -> w241
                tunnel: w240 -> [w348]
                shift-right: [w347] -> w232
                shift-left: w243 -> [w352]
                i -> [w344]
                stop <- w346 stop-if-true
                n127 = Increment(x=w344) -> (x+1=→"Image Acq 2":i32)
                n128 = call <userlib>:"AT Wait Buffer A.vi"("error in (no error)"=w352, "Timeout"=u32 11000, "Handle"=w350) -> ("error out"=w349:errorcluster, "Output buffer"=w351:u64)  [unwired: 5 in, 2 out]
                n129 = case shown="No Error" w349 {
                  selector: w349 -> [w355 w364]
                  tunnel: w351 -> [w357 _]
                  tunnel: [w354 w364] -> w347
                  tunnel: w348 -> [w356 _]
                  frame No Error {
                    n130 = local read "image pointers 2"() -> (w361:u64[])
                    n131 = Enqueue Element(queue=w356, element=w357, error in (no error)=w355) -> (error out=w354:errorcluster)  [unwired: 1 in, 2 out]
                    n132 = local read "count 2"() -> (w363:i32)
                    n133 = local read "imageNo 2"() -> (w358:i32)
                    n134 = Increment(x=w363) -> (x+1=w362:i32)
                    n135 = Insert Into Array(array=w361, index=w358, new element=w357) -> (w360:u64[])
                    n136 = Increment(x=w358) -> (x+1=w359:i32)
                    n137 = local write "count 2"(w362) -> ()
                    n138 = local write "imageNo 2"(w359) -> ()
                    n139 = local write "image pointers 2"(w360) -> ()
                  }
                  frame Error {
                  }
                }
                n140 = local read "Break"() -> (w346:bool)
              }
            }
            frame #1 {
              n141 = local write "Image SSD Saving 2"(w365) -> ()
              n142 = call <userlib>:"AT Command A.vi"("Feature"="AcquisitionStop" ("Command"), "Handle"=w367) -> ()  [unwired: 8 in, 2 out]
            }
            frame #2 {
              n143 = call <userlib>:"AT Flush A.vi"("Handle"=w373) -> ()  [unwired: 9 in, 2 out]
              n144 = call <userlib>:"AT Clear All Buffers A.vi"("Handle"=w373) -> ("error out"=w372:errorcluster)  [unwired: 9 in, 1 out]
              n145 = Merge Errors(w372, w374) -> (w375:errorcluster)
            }
          }
          n146 = Release Queue(queue=w202, error in (no error)=w199) -> (error out=w203:errorcluster)  [unwired: 1 in, 2 out]
          n147 = Merge Errors(w203, w198) -> (w213:errorcluster)
          "error dequeue 2" <- w198
        }
        frame condition #1 {
        }
      }
      n148 = flat-sequence {
        tunnel: [w433] -> w108
        tunnel: w65 -> [w433]
        tunnel: [w432] -> w72
        frame #0 {
          n149 = Get Date/Time In Seconds() -> (seconds since 1Jan1904=w432:timestamp)
        }
      }
      n150 = flat-sequence {
        tunnel: w105 -> [w459]
        tunnel: w14 -> [w437]
        tunnel: w68 -> [w458]
        tunnel: [w457] -> w115
        tunnel: [w452] -> w114
        tunnel: w62 -> [w454]
        tunnel: [w453] -> w107
        tunnel: w21 -> [w456]
        tunnel: w104 -> [w448]
        tunnel: [w455] -> w102
        tunnel: [w451] -> w95
        tunnel: w48 -> [w450]
        tunnel: [w447] -> w47
        tunnel: [w446] -> w45
        tunnel: w13 -> [w441]
        tunnel: w20 -> [w440]
        tunnel: w19 -> [w439]
        tunnel: w16 -> [w438]
        tunnel: w15 -> [w436]
        tunnel: w11 -> [w435]
        tunnel: w12 -> [w434]
        tunnel: w115 -> [w613]
        tunnel: w114 -> [w612]
        tunnel: w107 -> [w616]
        tunnel: w102 -> [w615]
        tunnel: w95 -> [w614]
        tunnel: [w613] -> w82
        tunnel: [w616] -> w81
        tunnel: [w615] -> w80
        tunnel: [w614] -> w79
        tunnel: [w612] -> w78
        tunnel: w47 -> [w611]
        tunnel: [w611] -> w46
        tunnel: w45 -> [w610]
        tunnel: [w610] -> w44
        tunnel: [w624] -> w69
        tunnel: [w625] -> w101
        tunnel: [w626] -> w99
        tunnel: [w623] -> w100
        tunnel: w82 -> [w621]
        tunnel: w81 -> [w626]
        tunnel: w80 -> [w625]
        tunnel: w79 -> [w624]
        tunnel: w78 -> [w622]
        tunnel: w46 -> [w619]
        tunnel: [w619] -> w41
        tunnel: w44 -> [w618]
        tunnel: [w618] -> w43
        frame #0 {
          n151 = for {
            N: w436 -> [_]
            tunnel: w454 -> [w473] mode=indexing
            tunnel: [w472] -> w453 mode=indexing
            tunnel: w439 -> [w463]
            shift-right: [w471] -> w447
            shift-left: errorcluster {"status"=FALSE, "code"=0, "source"=""} ("error out") -> [w470]
            tunnel: w440 -> [w469]
            tunnel: [w468] -> w446
            shift-right: [w467] -> w443
            shift-left: 0 -> [w466]
            tunnel: w441 -> [w464]
            tunnel: w438 -> [w462]
            tunnel: w435 -> [w461]
            tunnel: w434 -> [w460]
            stop <- w465 stop-if-true
            n152 = for {
              N: w461 -> [_]
              tunnel: w463 -> [w495]
              shift-right: [w493] -> w471
              shift-left: w470 -> [w488]
              shift-right: [w492] -> w467
              shift-left: w466 -> [w491]
              tunnel: w473 -> [w497]
              tunnel: [w496] -> w472
              tunnel: w469 -> [w487]
              tunnel: [w486] -> w468
              tunnel: w464 -> [w489]
              tunnel: w463 -> [w481]
              tunnel: w462 -> [w475]
              tunnel: w460 -> [w474]
              stop <- w490 stop-if-true
              n153 = for {
                N: w474 -> [_]
                shift-right: [w509] -> w480
                shift-left: w489 -> [w529]
                shift-right: [w525] -> w479
                shift-left: w489 -> [w528]
                shift-right: [w524] -> w478
                shift-left: w489 -> [w527]
                shift-right: [w523] -> w477
                shift-left: w489 -> [w526]
                shift-right: [w515] -> w485
                shift-left: w488 -> [w522]
                tunnel: w487 -> [w521]
                tunnel: [w514] -> w486
                tunnel: [w511] -> w483 mode=indexing
                tunnel: w481 -> [w508]
                tunnel: w475 -> [w505]
                i -> [w530]
                stop <- w498 stop-if-true
                n154 = Dequeue Element(queue=w521, timeout in ms (-1)=T17 11000 ("timeout for deque loop"), error in (no error)=w522) -> (queue out=w517:refnum<queue>, element=w506:u8[], timed out?=w507:bool, error out=w518:errorcluster)
                n155 = Tick Count (ms)() -> (millisecond timer value=w502:u32)
                n156 = call "SCMP - Process Low Level Camera Data Into Image v2.vi"("PixelData (U16)"=w505, "Andor Cluster"=w508, "Input buffer"=w506, "error in (no error)"=w518, "Demo pic \n(Andor/SCMP)"=TRUE ("scmp demo pic")) -> ("Image (I32)"=w513:u32[][], "Timestamp"=w511:timestamp, "error out"=w516:errorcluster)  [unwired: 8 in]
                n157 = Quotient & Remainder(x=w530, y=4) -> (x-y*floor(x/y)=w531:i32)  [unwired: 1 out]
                n158 = feedback #1(u32 0) -> (w503:u32)
                n159 = Greater?(x=w502, y=w503) -> (0:w510:bool)
                "display refresh" <- w510
                n160 = Add(x=u32 1200 ("y"), y=w502) -> (x+y=w504:u32)
                n161 = feedback-in #1(w504) -> ()
                n162 = case shown="0, Default" w531 {
                  tunnel: w526 -> [w539 w546 w552 w555]
                  tunnel: w527 -> [w540 w547 w549 w558]
                  tunnel: w528 -> [w541 w543 w553 w559]
                  tunnel: w529 -> [w537 w544 w550 w556]
                  tunnel: [w536 w544 w550 w556] -> w509
                  tunnel: [w541 w542 w553 w559] -> w525
                  tunnel: [w540 w547 w548 w558] -> w524
                  tunnel: [w539 w546 w552 w554] -> w523
                  tunnel: w513 -> [w538 w545 w551 w557]
                  frame 0, Default {
                    n163 = Add(x=w537, y=w538) -> (x+y=w536:u32[][])
                  }
                  frame 1 {
                    n164 = Add(x=w543, y=w545) -> (x+y=w542:u32[][])
                  }
                  frame 2 {
                    n165 = Add(x=w549, y=w551) -> (x+y=w548:u32[][])
                  }
                  frame 3 {
                    n166 = Add(x=w555, y=w557) -> (x+y=w554:u32[][])
                  }
                }
                n167 = Get Queue Status(queue=w517, error in (no error)=w516) -> (queue out=w514:refnum<queue>, error out=w515:errorcluster, # elements in queue=→"# elements in RAM queue":i32)  [unwired: 1 in, 5 out]
                n168 = case shown="True" w510 {
                  tunnel: w509 -> [_ w533]
                  frame False {
                  }
                  frame True {
                    n169 = disable-structure shown="SCMP==COMP, Default" {
                      disable-tunnel: w533 -> [w534 w535]
                      frame condition #0 (active) {
                        "Camera T Image wide" <- w534
                        "Camera T Image" <- w534
                      }
                      frame condition #1 {
                        "Image Cam" <- w535
                      }
                    }
                    "Image" <- w533
                  }
                }
                n170 = Or(x="user break", y=w507) -> (x .or. y?=w498:bool)
                "Break" <- w498
              }
              n171 = Build Array(w480, w479, w478, w477) -> (w476:u32[][][])
              n172 = Array Subset(array=w483, length=4) -> (w482:timestamp[])  [unwired: 1 in]
              "Time stamp arr" <- w482
              n173 = disable-structure shown="Disabled" {
                frame Disabled {
                  n174 = call "SCMP - picture flip rotate.vi"() -> ()  [unwired: 8 in, 4 out]
                }
                frame Enabled {
                }
              }
              n175 = Bundle By Name(cluster=w497, "Time Stamp Array"=w482) -> (w496:T12)
              n176 = case shown="True" "Save to FITS?" {
                tunnel: w496 -> [_ w568]
                tunnel: w495 -> [_ w567]
                tunnel: w491 -> [_ w566]
                tunnel: [w560 w563] -> w493
                tunnel: w485 -> [w560 w562]
                tunnel: w476 -> [_ w561]
                frame False {
                }
                frame True {
                  n177 = call "SCMP - Write FITS File v2.vi"("FITS Header"=w568, "Andor"=w567, "Data"=w561, "error in"=w562, "Image #"=w566) -> ("FITS Path Out"=w564:path, "error out"=w563:errorcluster)  [unwired: 8 in, 1 out]
                  n178 = Equal To 0?(x=w566) -> (x = 0?=w565:bool)
                  n179 = case shown="True" w565 {
                    tunnel: w564 -> [_ w569]
                    frame False {
                    }
                    frame True {
                      "FITS Path Out" <- w569
                    }
                  }
                }
              }
              n180 = Increment(x=w491) -> (x+1=w492:i32)
              n181 = local read "Break"() -> (w490:bool)
              "Image SSD Saving" <- w491
            }
            n182 = local read "Break"() -> (w465:bool)
          }
          n183 = for "Loop which waits for and build up list of image pointers for processing" {
            N: w437 -> [_]
            tunnel: w458 -> [w596]
            tunnel: [w596] -> w457
            tunnel: w448 -> [w594]
            shift-right: [w593] -> w452
            shift-left: w459 -> [w598]
            i -> [w591]
            stop <- w592 stop-if-true
            n184 = Increment(x=w591) -> (x+1=→"Image Acq":i32)
            n185 = call <userlib>:"AT Wait Buffer A.vi"("error in (no error)"=w598, "Timeout"=T17 11000 ("timeout for deque loop"), "Handle"=w596) -> ("error out"=w595:errorcluster, "Output buffer"=w597:u64)  [unwired: 5 in, 2 out]
            n186 = case shown="No Error" w595 {
              selector: w595 -> [w600 w609]
              tunnel: w597 -> [w602 _]
              tunnel: [w599 w609] -> w593
              tunnel: w594 -> [w601 _]
              frame No Error {
                n187 = local read "image pointers"() -> (w606:u64[])
                n188 = Enqueue Element(queue=w601, element=w602, error in (no error)=w600) -> (error out=w599:errorcluster)  [unwired: 1 in, 2 out]
                n189 = local read "count"() -> (w608:i32)
                n190 = local read "imageNo"() -> (w603:i32)
                n191 = Increment(x=w608) -> (x+1=w607:i32)
                n192 = Insert Into Array(array=w606, index=w603, new element=w602) -> (w605:u64[])
                n193 = Increment(x=w603) -> (x+1=w604:i32)
                n194 = local write "count"(w607) -> ()
                n195 = local write "imageNo"(w604) -> ()
                n196 = local write "image pointers"(w605) -> ()
              }
              frame Error {
              }
            }
            n197 = local read "Break"() -> (w592:bool)
          }
          n198 = for {
            N: w437 -> [_]
            tunnel: w456 -> [w587]
            shift-right: [w582] -> w451
            shift-left: w450 -> [w585]
            tunnel: w448 -> [w588]
            tunnel: [w586] -> w455
            tunnel: w440 -> [w581]
            shift-right: [w573] -> w442
            shift-left: u32 0 ("Image transfering") -> [w574]
            stop <- w584 stop-if-true
            n199 = Dequeue Element(queue=w588, timeout in ms (-1)=T17 11000 ("timeout for deque loop"), error in (no error)=w585) -> (queue out=w580:refnum<queue>, element=w577:u64, timed out?=w570:bool, error out=w576:errorcluster)
            n200 = Increment(x=w574) -> (x+1=w573:u32)
            n201 = local read "Break"() -> (w571:bool)
            n202 = call <userlib>:"PointerToArray.vi"("error in (no error)"=w576, "Pointer In"=w577, "Array in"=w587) -> ("error out"=w575:errorcluster, "Array out"=w572:u8[])  [unwired: 7 in]
            n203 = Or(x=w571, y=w570) -> (x .or. y?=w584:bool)
            n204 = Get Queue Status(queue=w580, error in (no error)=w575) -> (queue out=w586:refnum<queue>, error out=w583:errorcluster, # elements in queue=→"# elements in queue":i32)  [unwired: 1 in, 5 out]
            n205 = Enqueue Element(queue=w581, element=w572, error in (no error)=w583) -> (error out=w582:errorcluster)  [unwired: 1 in, 2 out]
            "Image transfering" <- w574
          }
          n206 = local write "Image transfering"(w442) -> ()
          n207 = local write "Image SSD Saving"(w443) -> ()
        }
        frame #1 {
          n208 = call <userlib>:"AT Command A.vi"("Feature"="AcquisitionStop" ("Command"), "Handle"=w613) -> ()  [unwired: 8 in, 2 out]
        }
        frame #2 {
          n209 = call <userlib>:"AT Flush A.vi"("Handle"=w621) -> ()  [unwired: 9 in, 2 out]
          n210 = call <userlib>:"AT Clear All Buffers A.vi"("Handle"=w621) -> ("error out"=w620:errorcluster)  [unwired: 9 in, 1 out]
          n211 = Merge Errors(w620, w622) -> (w623:errorcluster)
        }
      }
      n212 = call "SCD - Timestamp AO Waveform.vi"("DAQ To"=w72, "SCD AO Waveforms"=w97) -> ()  [unwired: 8 in, 2 out]
      n213 = call <vilib>:"DAQmx Start Task.vi"("task/channels in"=w67, "error in"=w108) -> ("task out"=w131:refnum<k21>, "error out"=w51:errorcluster)  [unwired: 12 in]
      n214 = call "PDSS - Turn Trigger Light On.vi"("error in (no error)"=w51) -> ("error out"=w123:errorcluster, "Trigger Started"=→"Image Acq Started":bool)  [unwired: 9 in]
      n215 = Multiply(x=1000.0, y=w34) -> (x*y=w52:dbl)
      n216 = disable-structure shown="Disabled" {
        disable-tunnel: w131 -> [w143 w145]
        disable-tunnel: w123 -> [w142 w144]
        disable-tunnel: [w140 w144] -> w36
        disable-tunnel: w34 -> [w138 _]
        disable-tunnel: [_ w145] -> w33
        frame Disabled {
          n217 = Multiply(x=w138, y=1.25 ("x")) -> (x*y=w141:dbl)
          n218 = call <vilib>:"DAQmx Wait Until Done.vi"("task/channels in"=w143, "timeout (sec)"=w141, "error in"=w142) -> ("error out"=w140:errorcluster)  [unwired: 11 in, 1 out]
        }
        frame Enabled {
        }
      }
      n219 = property on="Image Acq (s)" class="Slide (strict)"(error in=w51, "Scale.Maximum"=w52) -> (error out=w50:errorcluster)  [unwired: 1 in, 1 out]
      n220 = while {
        tunnel: w52 -> [w165]
        tunnel: w50 -> [_]
        tunnel: w36 -> [w169]
        tunnel: [w168] -> w35
        tunnel: w33 -> [w167]
        tunnel: [w166] -> w32
        tunnel: [w164] -> w30
        i -> [w171]
        stop <- w161 stop-if-true
        w170 = u32 300 ("milliseconds to wait")
        n221 = Multiply(x=w171, y=w170) -> (x*y=w172:u32)
        n222 = Wait (ms)(milliseconds to wait=w170) -> ()  [unwired: 1 out]
        n223 = Subtract(x=w165, y=w172) -> (x-y=w164:dbl)
        "Image Acq (s)" <- w164
        n224 = call <vilib>:"DAQmx Is Task Done.vi"("task/channels in"=w167, "error in"=w169) -> ("task out"=w166:refnum<k21>, "task done?"=w163:bool, "error out"=w168:errorcluster)  [unwired: 11 in]
        n225 = local read "Break 2"() -> (w160:bool)
        n226 = local read "Break"() -> (w162:bool)
        n227 = Compound Arithmetic op=OR(w160, w162, w163) -> (w161:bool)
      }
      n228 = Multiply(x=w30, y=0.0 ("Image Acq (s)")) -> (x*y=w29:dbl)
      n229 = call <vilib>:"DAQmx Stop Task.vi"("task/channels in"=w32, "error in"=w35) -> ("task out"=w130:refnum<k21>, "error out"=w129:errorcluster)  [unwired: 12 in]
      n230 = local write "Image Acq (s)"(w29) -> ()
      n231 = call <vilib>:"DAQmx Clear Task.vi"("task in"=w130, "error in"=w129) -> ("error out"=w118:errorcluster)  [unwired: 13 in]
      n232 = invoke on="Image Acq Started" class="Bool (strict)" method="Reinit To Default"(error in=w118) -> (error out=w117:errorcluster)  [unwired: 2 in, 2 out]
      n233 = disable-structure shown="SCMP==SCD" {
        disable-tunnel: [tag "PXI-6733/port0/line0" ("lines") tag "Dev3/port0/line0" ("comp lines")] -> w94
        disable-tunnel: [tag "PXI-6733/ao0:7" ("physical channels") tag "Dev3/ao0:7" ("physical channels")] -> w93
        frame condition #0 {
        }
        frame condition #1 (active) {
        }
      }
      n234 = call "SCD - Trigger Sequence - Set All AO Values to Zero.vi"("error in"=w117, "lines"=w94, "physical channels"=w93) -> ("error out"=w112:errorcluster)  [unwired: 8 in]
      n235 = global read "Global demo.vi" "demo"() -> (w27:bool)
      n236 = Release Queue(queue=w43, error in (no error)=w41) -> (error out=w42:errorcluster)  [unwired: 1 in, 2 out]
      n237 = Release Queue(queue=w101, error in (no error)=w100) -> (error out=w96:errorcluster)  [unwired: 1 in, 2 out]
      n238 = Merge Errors(w61, w96, w69, w42) -> (w31:errorcluster)
      n239 = case shown="True" w27 {
        tunnel: w31 -> [_ _]
        frame False {
        }
        frame True {
          # "len ukoncenie daq slucky\n v demo mode skor"
          "Break 2" <- TRUE ("Break 2")
        }
      }
      n240 = Merge Errors(w31, w112) -> (w111:errorcluster)
      "Headers Out" <- w99
      "error cam dequeue & queue RAM" <- w69
      "Time Start" <- w72
      "error dequeue RAM" <- w41
    }
    frame Error {
    }
  }
  "error out" <- w9
  n241 = disable-structure shown="Disabled" {
    frame Disabled {
      # "someday this\nmight speed up\naccumulatons"
      n242 = call "SCD - Extract Image Vector and Timestamp from Pointer.vi"() -> ()  [unwired: 13 in, 3 out]
    }
    frame Enabled {
    }
  }
